vi "DBAL-Service.vi"(8 "error in (no error)":errorcluster, 11 "DBAL_in":refnum<class "DBAL.lvclass">) -> (0 "error out":errorcluster, 3 "DBAL_out":refnum<class "DBAL.lvclass">)   [LabVIEW 2020, in "Sgraph_lib_V1.lvlib" / "DBAL.lvclass"]
uses:
  DBAL.lvclass
  DBAL.lvclass/DBAL.ctl
panel:
  out "Saved data":T1(array[cluster])
  out "37x37":picture
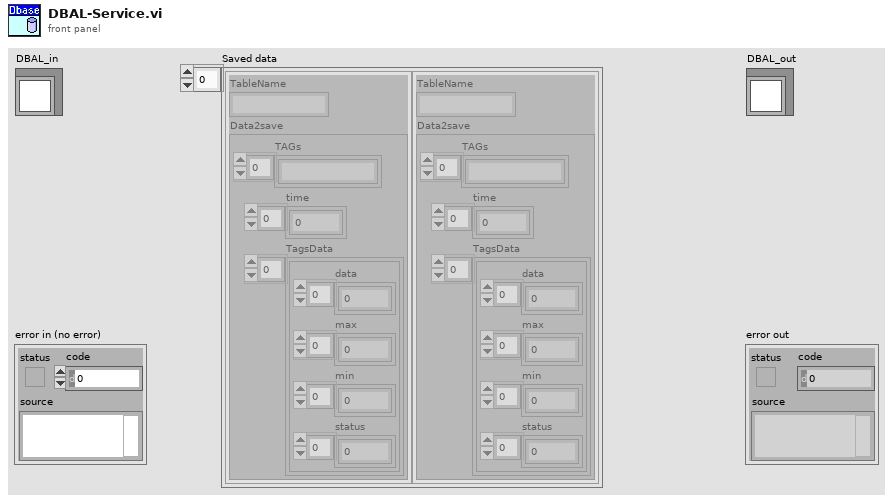
[diagram p1: front panel]
types:
  T1 = cluster{"TableName":string, "Data2save":cluster{"TAGs":string[], "time":dbl[], "TagsData":cluster{"data":dbl[], "max":dbl[], "min":dbl[], "status":u32[]}[]}}[]
  T2 = typedef "Sgraph_lib_V1.lvlib/DBAL.lvclass/DBAL_Command.ctl" = cluster{"Source":string, "Command":T3, "Time Stamp":timestamp, "data":variant}
  T3 = typedef "Sgraph_lib_V1.lvlib/DBAL.lvclass/DBAL-commands.ctl" = enum16{"idle", "SavePAQdata", "ExitService"}
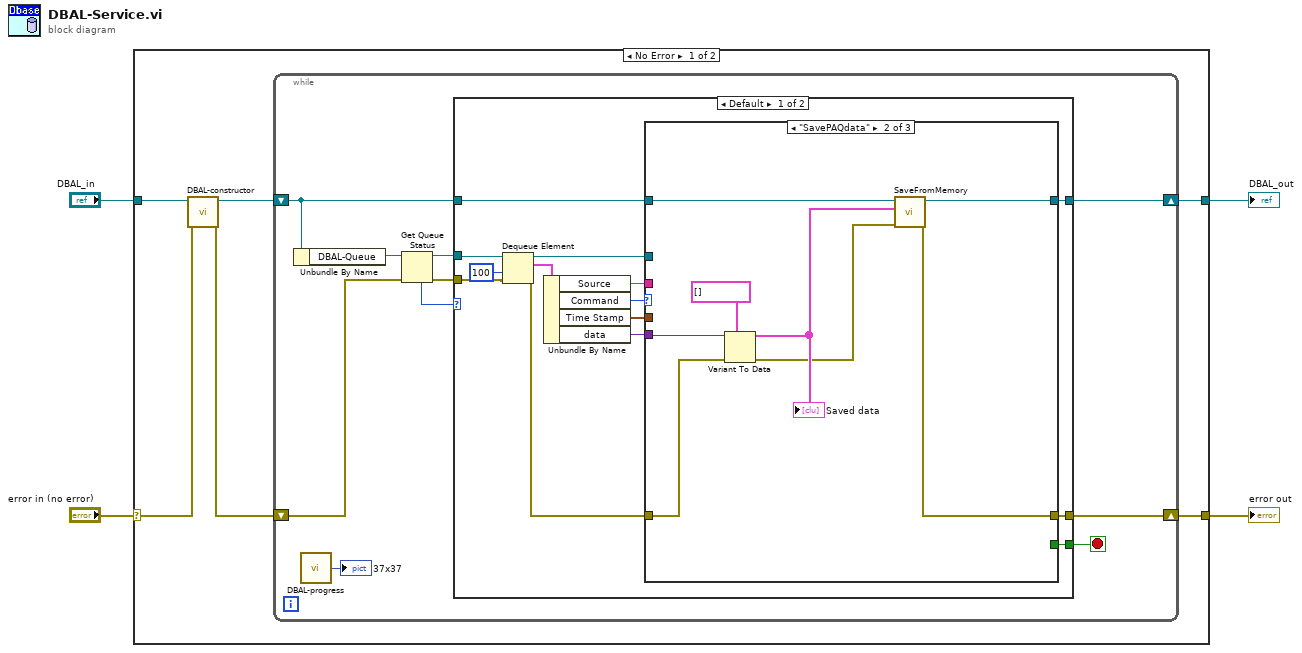
[diagram p0: block diagram]
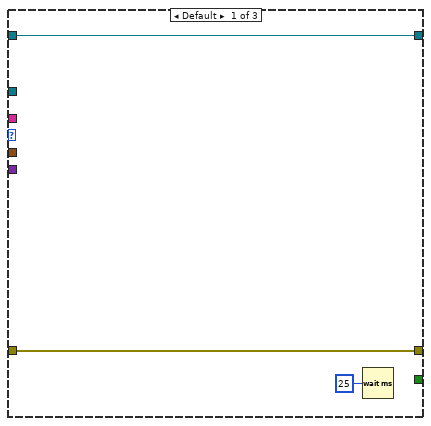
[diagram p2: hidden frame]
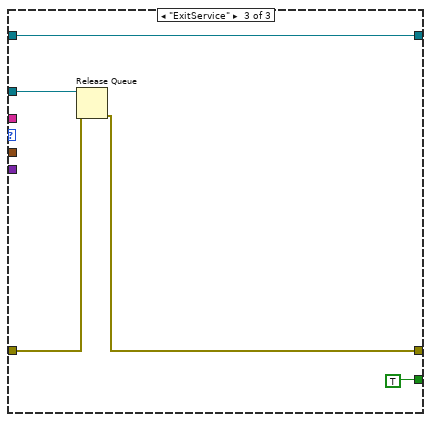
[diagram p3: hidden frame]
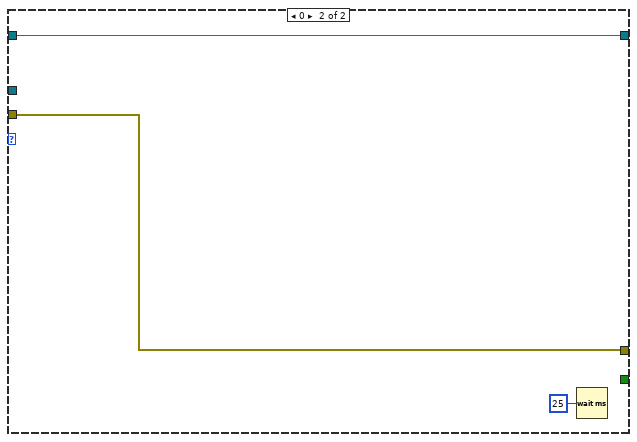
[diagram p4: hidden frame]
diagram:
  n1 = case shown="No Error" "error in (no error)" {
    selector: "error in (no error)" -> [w6 w55]
    tunnel: [w9 w55] -> w3
    tunnel: [w10 w54] -> w1
    tunnel: "DBAL_in" -> [w7 w54]
    frame No Error {
      n2 = call "DBAL-constructor.vi"("error in (no error)"=w6, "DBAL in"=w7) -> ("error out"=w5:errorcluster, "DBAL out"=w8:refnum<class "DBAL.lvclass">)  [unwired: 8 in]
      n3 = while {
        shift-right: [w16] -> w10
        shift-left: w8 -> [w17]
        shift-right: [w12] -> w9
        shift-left: w5 -> [w14]
        stop <- w11 stop-if-true
        n4 = Unbundle By Name(w17) -> ("DBAL-Queue"=w19:refnum<queue>)
        n5 = call "DBAL-progress.vi"() -> ("37x37"=→"37x37":picture)  [unwired: 7 in]
        n6 = Get Queue Status(queue=w19, error in (no error)=w14) -> (queue out=w15:refnum<queue>, error out=w13:errorcluster, # elements in queue=w18:i32)  [unwired: 1 in, 5 out]
        n7 = case shown="Default" w18 {
          tunnel: w17 -> [w26 w53]
          tunnel: [w25 w53] -> w16
          tunnel: w15 -> [w34 _]
          tunnel: w13 -> [w32 w52]
          tunnel: [w23 w52] -> w12
          tunnel: [w22 _] -> w11
          frame Default {
            n8 = Dequeue Element(queue=w34, timeout in ms (-1)=100, error in (no error)=w32) -> (queue out=w21:refnum<queue>, element=w31:T2, error out=w24:errorcluster)  [unwired: 1 out]
            n9 = Unbundle By Name(w31) -> ("Source"=w27:string, "Command"=w30:T3, "Time Stamp"=w29:timestamp, "data"=w28:variant)
            n10 = case shown="\"SavePAQdata\"" w30 {
              tunnel: w29 -> [_ _ _]
              tunnel: w28 -> [_ w42 _]
              tunnel: w27 -> [_ _ _]
              tunnel: w26 -> [w37 w44 w50]
              tunnel: [w37 w45 w50] -> w25
              tunnel: w24 -> [w36 w38 w46]
              tunnel: [w36 w43 w47] -> w23
              tunnel: [_ _ TRUE] -> w22
              tunnel: w21 -> [_ _ w48]
              frame Default {
                n11 = Wait (ms)(milliseconds to wait=u32 25) -> ()  [unwired: 1 out]
              }
              frame "SavePAQdata" {
                n12 = Variant To Data(error in=w38, type=T1 [] ("Data_2_Save"), Variant=w42) -> (data=w40:T1, error out=w39:errorcluster)
                "Saved data" <- w40
                n13 = call-dynamic "SaveFromMemory.vi"("error in (no error)"=w39, "Data_2_Save"=w40, "DBAL in"=w44) -> ("error out"=w43:errorcluster, "DBAL out"=w45:refnum<class "DBAL.lvclass">)  [unwired: 7 in]
              }
              frame "ExitService" {
                n14 = Release Queue(queue=w48, error in (no error)=w46) -> (error out=w47:errorcluster)  [unwired: 1 in, 2 out]
              }
            }
          }
          frame 0 {
            n15 = Wait (ms)(milliseconds to wait=u32 25) -> ()  [unwired: 1 out]
          }
        }
      }
    }
    frame Error {
    }
  }
  "error out" <- w3
  "DBAL_out" <- w1
